vi "Lab Panel V6.00.vi"() -> ()   [LabVIEW 2017]
uses:
  sub vi/TEmp Indicator.ctl
  sub vi/SelectLAB0X-N.ctl
  sub vi/SIG LAB0X-N.ctl
  sub vi/Set LAB0X-N.ctl
  sub vi/Disp Lab.ctl
  TEmp.ctl
  <vilib>/Platform/TimedLoop/XDataNode/timing_clust.ctl
  <vilib>/Platform/TimedLoop/XDataNode/nitl_modes.ctl
  <vilib>/Platform/TimedLoop/XDataNode/wakeup.ctl
  Global 1.vi
  Global display 4.vi
  Global display 3.vi
  Global display 1.vi
  Global display 2.vi
  <vilib>/platform/TimedLoop/XDataNode/XDataNode.xnode
  <vilib>/Platform/TimedLoop/XDataNode/XDNodeRunTimeDep.lvlib
  sub vi/Web Imge control.ctl
panel:
  in  "path to JPEG file":path=path "C:/Users/Mike/Documents/Crabtree/Crabtree/Hardware/crabtree"
  out "Simulate IND":bool
  out "network error":bool
  out "TEMP":bool
  out "AI":bool
  out "Amb Temp":dbl format="%#.0f"
  out "Temp Up":dbl
  in  "stop all":bool
  in  "ADMIN":bool
  in  "Tab Control 2":T1(tab)
  out "SIG LAB05-2":T2 {"PF" format="%.2f"; "AMPS" format="%.1f"}
  out "SIG LAB05-1":T2 {"PF" format="%.2f"; "AMPS" format="%.1f"}
  out "SIG LAB04-2":T2 {"PF" format="%.2f"; "AMPS" format="%.1f"}
  out "SIG LAB04-1":T2 {"PF" format="%.2f"; "AMPS" format="%.1f"}
  out "SIG LAB03-2":T2 {"PF" format="%.2f"; "AMPS" format="%.1f"}
  out "SIG LAB03-1":T2 {"PF" format="%.2f"; "AMPS" format="%.1f"}
  out "SIG LAB02-2":T2 {"PF" format="%.2f"; "AMPS" format="%.1f"}
  in  "RUN LAB01-1":bool
  in  "O/I  LAB05-1":bool
  in  "O/I  LAB05-2":bool
  in  "O/I  LAB04-1":bool
  in  "O/I  LAB04-2":bool
  in  "O/I  LAB02-1":bool
  in  "O/I  LAB02-2":bool
  in  "O/I  LAB01-2":bool
  in  "O/I  LAB01-1":bool
  in  "O/I  LAB03-1":bool
  in  "RUN LAB05-2":bool
  in  "RUN LAB05-1":bool
  in  "RUN LAB04-2":bool
  in  "RUN LAB04-1":bool
  in  "RUN LAB03-2":bool
  in  "RUN LAB03-1":bool
  in  "RUN LAB02-2":bool
  in  "RUN LAB02-1":bool
  in  "RUN LAB01-2":bool
  in  "SELECT LAB05-2":T3
  in  "SELECT LAB05-1":T3
  in  "SELECT LAB04-2":T3
  in  "SELECT LAB04-1":T3
  in  "SELECT LAB03-2":T3
  in  "SELECT LAB03-1":T3
  in  "SELECT LAB02-2":T3
  in  "SELECT LAB02-1":T3
  in  "SELECT LAB01-2":T3
  in  "SELECT LAB01-1":T3
  in  "O/I  LAB03-2":bool
  out "SIG LAB01-1":T2 {"PF" format="%.2f"; "AMPS" format="%.1f"}
  out "SIG LAB01-2":T2 {"PF" format="%.2f"; "AMPS" format="%.1f"}
  out "SIG LAB02-1":T2 {"PF" format="%.2f"; "AMPS" format="%.1f"}
  out "DISP LAB05-2":T4 {"MINS" format="%.2g"}
  out "DISP LAB05-1":T4 {"MINS" format="%.2g"}
  out "DISP LAB04-2":T4 {"MINS" format="%.2g"}
  out "DISP LAB04-1":T4 {"MINS" format="%.2g"}
  out "DISP LAB03-2":T4 {"MINS" format="%.2g"}
  out "DISP LAB03-1":T4 {"MINS" format="%.2g"}
  in  "SET LAB05-2":T5={"NAME"="", "DESCRIPTION"="", "CYCLES"=5.0, "T-RISE mins"=0.0, "T-RISE deg C"=0.0} {"CYCLES" min=5.0 step=1.0}
  in  "SET LAB05-1":T5={"NAME"="", "DESCRIPTION"="", "CYCLES"=5.0, "T-RISE mins"=0.0, "T-RISE deg C"=0.0} {"CYCLES" min=5.0 step=1.0}
  in  "SET LAB04-2":T5={"NAME"="", "DESCRIPTION"="", "CYCLES"=5.0, "T-RISE mins"=0.0, "T-RISE deg C"=0.0} {"CYCLES" min=5.0 step=1.0}
  in  "SET LAB04-1":T5={"NAME"="", "DESCRIPTION"="", "CYCLES"=5.0, "T-RISE mins"=0.0, "T-RISE deg C"=0.0} {"CYCLES" min=5.0 step=1.0}
  in  "SET LAB03-2":T5={"NAME"="", "DESCRIPTION"="", "CYCLES"=5.0, "T-RISE mins"=0.0, "T-RISE deg C"=0.0} {"CYCLES" min=5.0 step=1.0}
  in  "SET LAB03-1":T5={"NAME"="", "DESCRIPTION"="", "CYCLES"=5.0, "T-RISE mins"=0.0, "T-RISE deg C"=0.0} {"CYCLES" min=5.0 step=1.0}
  out "DISP LAB02-2":T4 {"MINS" format="%.2g"}
  out "DISP LAB02-1":T4 {"MINS" format="%.2g"}
  in  "SET LAB02-2":T5={"NAME"="", "DESCRIPTION"="", "CYCLES"=5.0, "T-RISE mins"=0.0, "T-RISE deg C"=0.0} {"CYCLES" min=5.0 step=1.0}
  in  "SET LAB02-1":T5={"NAME"="", "DESCRIPTION"="", "CYCLES"=5.0, "T-RISE mins"=0.0, "T-RISE deg C"=0.0} {"CYCLES" min=5.0 step=1.0}
  out "RESULT LAB05-2":bool
  out "RESULT LAB05-1":bool
  out "RESULT LAB04-2":bool
  out "RESULT LAB04-1":bool
  out "RESULT LAB03-2":bool
  out "RESULT LAB03-1":bool
  out "RESULT LAB02-2":bool
  out "RESULT LAB02-1":bool
  out "RESULT LAB01-2":bool
  out "RESULT LAB01-1":bool
  in  "SET LAB01-1":T5={"NAME"="", "DESCRIPTION"="", "CYCLES"=5.0, "T-RISE mins"=0.0, "T-RISE deg C"=0.0} {"CYCLES" min=5.0 step=1.0}
  in  "SET LAB01-2":T5={"NAME"="", "DESCRIPTION"="", "CYCLES"=5.0, "T-RISE mins"=0.0, "T-RISE deg C"=0.0} {"CYCLES" min=5.0 step=1.0}
  out "DISP LAB01-1":T4 {"MINS" format="%.2g"}
  out "DISP LAB01-2":T4 {"MINS" format="%.2g"}
  out "TEMP RISE LAB05-2":cluster{"TL":dbl, "TN":dbl}
  out "TEMP RISE LAB05-1":cluster{"TL":dbl, "TN":dbl}
  out "TEMP RISE LAB04-2":cluster{"TL":dbl, "TN":dbl}
  out "TEMP RISE LAB04-1":cluster{"TL":dbl, "TN":dbl}
  out "TEMP RISE LAB03-2":cluster{"TL":dbl, "TN":dbl}
  out "TEMP RISE LAB03-1":cluster{"TL":dbl, "TN":dbl}
  out "TEMP RISE LAB02-2":cluster{"TL":dbl, "TN":dbl}
  out "TEMP RISE LAB02-1":cluster{"TL":dbl, "TN":dbl}
  out "TEMP RISE LAB01-2":cluster{"TL":dbl, "TN":dbl}
  out "TEMP RISE LAB01-1":cluster{"TL":dbl, "TN":dbl}
  out "JIG LAB05-2":bool
  out "JIG LAB05-1":bool
  out "JIG LAB04-2":bool
  out "JIG LAB04-1":bool
  out "JIG LAB03-2":bool
  out "JIG LAB03-1":bool
  out "JIG LAB02-2":bool
  out "JIG LAB02-1":bool
  out "JIG LAB01-2":bool
  out "JIG LAB01-1":bool
  out "TEMP START LAB01-1":cluster{"TL":dbl, "TN":dbl}
  out "TEMP START LAB02-1":cluster{"TL":dbl, "TN":dbl}
  out "TEMP START LAB03-1":cluster{"TL":dbl, "TN":dbl}
  out "TEMP START LAB04-1":cluster{"TL":dbl, "TN":dbl}
  out "TEMP START LAB01-2":cluster{"TL":dbl, "TN":dbl}
  out "TEMP START LAB02-2":cluster{"TL":dbl, "TN":dbl}
  out "TEMP START LAB03-2":cluster{"TL":dbl, "TN":dbl}
  out "TEMP START LAB04-2":cluster{"TL":dbl, "TN":dbl}
  out "TEMP START LAB05-2":cluster{"TL":dbl, "TN":dbl}
  out "TEMP START LAB05-1":cluster{"TL":dbl, "TN":dbl}
  out "LOG LAB05-2":string
  out "LOG LAB04-2":string
  out "LOG LAB03-2":string
  out "LOG LAB02-2":string
  out "LOG LAB01-2":string
  out "LOG LAB05-1":string
  out "LOG LAB04-1":string
  out "LOG LAB03-1":string
  out "LOG LAB02-1":string
  out "LOG LAB01-1":string
  in  "Tab charts":T6(tab)
  out "LAB01 VOLTS":dynamicdata(graph)
  out "LAB01 AMPS":dynamicdata(graph)
  out "LAB01 deg C":dynamicdata(graph)
  out "LAB02 VOLTS":dynamicdata(graph)
  out "LAB02 AMPS":dynamicdata(graph)
  out "LAB02 deg C":dynamicdata(graph)
  out "LAB03 VOLTS":dynamicdata(graph)
  out "LAB03 AMPS":dynamicdata(graph)
  out "LAB03 deg C":dynamicdata(graph)
  out "LAB04 VOLTS":dynamicdata(graph)
  out "LAB04 AMPS":dynamicdata(graph)
  out "LAB04 deg C":dynamicdata(graph)
  out "LAB05 VOLTS":dynamicdata(graph)
  out "LAB05 AMPS":dynamicdata(graph)
  out "LAB05 deg C":dynamicdata(graph)
  out "Reset Error":bool
  out "Er USB#2":dbl
  out "Er USB#1":dbl
  out "Er USB#0":dbl
  out "Resets Done":dbl
  out "Error USB #2":bool
  out "Error USB #1":bool
  out "Error USB #0":bool
  in  "MAIL SETTINGS":T7
  out "MAIL REPORT":string
  in  "TO (string):":string
  in  "Send Mail Now":bool
  in  "Auto Mail Send":bool
  in  "Network Directory":path
  in  "JIG ON TIME (S)":dbl=1.0 min=1.0 max=10.0 step=0.5 format="%.1g"
  in  "JIG OFF TIME (S)":dbl=2.0 min=2.0 max=10.0 step=0.5 format="%.1g"
  in  "Reset Measuring":bool
  out "path":path
  out "physical channels 0":string="DemoDevice,BID#0/ai0:1" caption="property value"
  out "physical channels 1":string="DemoDevice,BID#0/ai0:1" caption="property value"
  out "physical channels 2":string="DemoDevice,BID#0/ai0:1" caption="property value"
  in  "Min I":dbl=1.0
  in  "Min V":dbl=10.0
  out "JIG RELAY CYCLES":T8
  out "ON L05-2":cluster{"amps":dbl, "volts":dbl, "pf":dbl}
  out "ON L05-1":cluster{"amps":dbl, "volts":dbl, "pf":dbl}
  out "FAIL LAB05-2":cluster{"LO":dbl, "HI":dbl}
  out "FAIL LAB05-1":cluster{"LO":dbl, "HI":dbl}
  out "FAIL LAB04-2":cluster{"LO":dbl, "HI":dbl}
  out "FAIL LAB04-1":cluster{"LO":dbl, "HI":dbl}
  out "FAIL LAB03-2":cluster{"LO":dbl, "HI":dbl}
  out "FAIL LAB03-1":cluster{"LO":dbl, "HI":dbl}
  out "FAIL LAB02-2":cluster{"LO":dbl, "HI":dbl}
  out "FAIL LAB02-1":cluster{"LO":dbl, "HI":dbl}
  out "FAIL LAB01-2":cluster{"LO":dbl, "HI":dbl}
  out "FAIL LAB01-1":cluster{"LO":dbl, "HI":dbl}
  out "ON L01-1":cluster{"amps":dbl, "volts":dbl, "pf":dbl}
  out "ON L01-2":cluster{"amps":dbl, "volts":dbl, "pf":dbl}
  out "ON L02-1":cluster{"amps":dbl, "volts":dbl, "pf":dbl}
  out "ON L02-2":cluster{"amps":dbl, "volts":dbl, "pf":dbl}
  out "ON L03-1":cluster{"amps":dbl, "volts":dbl, "pf":dbl}
  out "ON L03-2":cluster{"amps":dbl, "volts":dbl, "pf":dbl}
  out "ON L04-1":cluster{"amps":dbl, "volts":dbl, "pf":dbl}
  out "ON L04-2":cluster{"amps":dbl, "volts":dbl, "pf":dbl}
  in  "Open Com Port":bool
  out "LA05-2 (TN)":bool
  out "LA05-2 (TL)":bool
  out "LA05-1 (TN)":bool
  out "LA05-1 (TL)":bool
  out "LA04-2 (TN)":bool
  out "LA04-2 (TL)":bool
  out "LA04-1 (TN)":bool
  out "LA04-1 (TL)":bool
  out "LA03-2 (TN)":bool
  out "LA03-2 (TL)":bool
  out "LA03-1 (TN)":bool
  out "LA03-1 (TL)":bool
  out "LA02-2 (TN)":bool
  out "LA02-2 (TL)":bool
  out "LA02-1 (TN)":bool
  out "LA02-1 (TL)":bool
  out "LA01-2 (TN)":bool
  out "LA01-2 (TL)":bool
  out "LA01-1 (TN)":bool
  out "LA01-1 (TL)":bool
  out "TEMP LA05":T9
  out "TEMP LA04":T9
  out "TEMP LA03":T9
  out "TEMP LA02":T9
  out "TEMP LA01":T9
  out "Ref deg C":dbl format="%#.0f"
  out "Temp read loop":dbl
  out "Com Port Status":bool
  out "Com setup loops":i32
  out "VISA Com out":refnum<visa-resource-name>
  in  "Select COM port":refnum<visa-resource-name>="COM6"
  in  "Read Temp":bool
  out "Error Temp":bool
  out "Fault Counters":u64[](array[numeric])
  out "TempErrors":bool[](array[boolean])
  in  "Temp Simulate":bool
  out "AI Task":bool
  out "AI Task2":u32
  out "AI Task1":u32
  out "AI Task0":u64
  out "Total USB resets":dbl
  in  "Auto Reset":bool
  in  "Mail Test File To:":string
  in  "Mail Test Fail":bool
  out "graph flag":bool
  in  "Temp Test Cal":dbl
  in  "Amps Fail level":dbl
  in  "Fail Loops":dbl
  out "Save JC":bool
  in  "DAQ Simulate":bool
  in  "Temp Value":dbl
  in  "Temp Delay Lps":dbl
  in  "SAMPLES":dbl
  in  "RATE (Hz)":dbl
  in  "JIG TEST":T10
  in  "C drive data root dir":path
  out "run lab05-2":bool
  out "run lab05-1":bool
  out "run lab04-2":bool
  out "run lab04-1":bool
  out "run lab03-2":bool
  out "run lab03-1":bool
  out "run lab02-2":bool
  out "run lab02-1":bool
  out "run lab01-2":bool
  out "run lab01-1":bool
  in  "Tab Control":T11(tab)
  out "LAB01-2 (GRAPH)":dynamicdata(graph)
  out "LAB01-1 (GRAPH)":dynamicdata(graph)
  out "LAB02-2 (GRAPH)":dynamicdata(graph)
  out "LAB02-1 (GRAPH)":dynamicdata(graph)
  out "LAB03-2 (GRAPH)":dynamicdata(graph)
  out "LAB03-1 (GRAPH)":dynamicdata(graph)
  out "LAB04-2 (GRAPH)":dynamicdata(graph)
  out "LAB04-1 (GRAPH)":dynamicdata(graph)
  out "LAB05-2 (GRAPH)":dynamicdata(graph)
  out "LAB05-1 (GRAPH)":dynamicdata(graph)
  out "Any Test Running":bool
  out "Read Time":dbl
  out "LAB05 TEMP":T12
  out "LAB04 TEMP":T12
  out "LAB02 TEMP":T12
  out "LAB01 TEMP":T12
  out "LAB03 TEMP":T12
  out "LAB05-TP":bool
  out "LAB04-TP":bool
  out "LAB03-TP":bool
  out "LAB02-TP":bool
  out "LAB01-TP":bool
  out "Analog error":bool
  out "USB OUT 0":bool[](array[boolean])
  out "USB OUT 1":bool[](array[boolean])
  out "USB OUT 2":bool[](array[boolean])
  in  "Ambient Volts":dbl format="%.2f"
  in  "PF":dbl min=0.0 max=1.0 step=0.1 format="%#.1f"
  in  "VOLTS":dbl
  in  "OFF amps":dbl min=0.0 max=100.0 step=0.1 format="%#.1f"
  in  "ON amps":dbl
  in  "LAB deg C":T13
  out "AI data 0":waveform(dbl)[](array[waveform])
  out "AI data 1":waveform(dbl)[](array[waveform])
  out "AI data 2":waveform(dbl)[](array[waveform])
  out "AI Error":errorcluster[](array[cluster])
  out "error array":errorcluster[](array[cluster])
  out "AI loop time":dbl format="%.6g"
  out "loops":dbl
  out "on loops":dbl format="%#.0f"
  out "off loops":dbl format="%#.0f"
  out "jig cycle":dbl
  out "TDMS LAB01-1":refnum<k34>
  out "data file error":errorcluster
  out "TDMS LAB02-1":refnum<k34>
  out "TDMS LAB01-2":refnum<k34>
  out "TDMS LAB02-2":refnum<k34>
  out "TDMS LAB03-1":refnum<k34>
  out "TDMS LAB03-2":refnum<k34>
  out "TDMS LAB04-1":refnum<k34>
  out "TDMS LAB04-2":refnum<k34>
  out "TDMS LAB05-1":refnum<k34>
  out "TDMS LAB05-2":refnum<k34>
  out "mail control":string
  out "File Time Stamp":timestamp
  in  "stop":bool
  out "deg C (volts)":dbl
  out "Application Directory":path
  out "ACQ Init TIme":u32
  out "ACQ Time":u32
  out "Web Server:Root Directory Path":path
  out "Analog Fault Counts":i32[](array[numeric])
  out "Timed loop Finished Late":bool
  in  "Set Loop Time":T14=500.0 format="%#_13g"
  out "Loop Time":u32
  out "Process AIs":bool
  in  "DigOutDelay":u32=5
  out "TEMP REF cal":dbl
  out "CAL LAB01":T15 {"2 (TN) cal" min=0.0 step=0.01 format="%.2f"; "2 (TL) cal" min=0.0 step=0.01 format="%.2f"; "2 (PF) cal" min=0.0 step=0.01 format="%.2f"; "2 (V) cal" min=0.0 step=0.01 format="%.2f"; "2 (A) cal" min=0.0 step=0.01 format="%.2f"; "1 (TN) cal" min=0.0 step=0.01 format="%.2f"; "1 (TL) cal" min=0.0 step=0.01 format="%.2f"; "1 (PF) cal" min=0.0 step=0.01 format="%.2f"; "1 (V) cal" min=0.0 step=0.01 format="%.2f"; "1  (A) cal" min=0.0 step=0.01 format="%.2f"}
  out "CAL LAB03":T15 {"2 (TN) cal" min=0.0 step=0.01 format="%.2f"; "2 (TL) cal" min=0.0 step=0.01 format="%.2f"; "2 (PF) cal" min=0.0 step=0.01 format="%.2f"; "2 (V) cal" min=0.0 step=0.01 format="%.2f"; "2 (A) cal" min=0.0 step=0.01 format="%.2f"; "1 (TN) cal" min=0.0 step=0.01 format="%.2f"; "1 (TL) cal" min=0.0 step=0.01 format="%.2f"; "1 (PF) cal" min=0.0 step=0.01 format="%.2f"; "1 (V) cal" min=0.0 step=0.01 format="%.2f"; "1  (A) cal" min=0.0 step=0.01 format="%.2f"}
  out "CAL LAB02":T16 {"2 (TN) cal" min=0.0 step=0.01 format="%.2f"; "2 (TL) cal" min=0.0 step=0.01 format="%.2f"; "2 (PF) cal" min=0.0 step=0.01 format="%.2f"; "2 (V) cal" min=0.0 step=0.01 format="%.2f"; "2 (A) cal" min=0.0 step=0.01 format="%.2f"; "1 (TN) cal" min=0.0 step=0.01 format="%.2f"; "1 (TL) cal" min=0.0 step=0.01 format="%.2f"; "1 (PF) cal" min=0.0 step=0.01 format="%.2f"; "1 (V) cal" min=0.0 step=0.01 format="%.2f"; "1 (A) cal" min=0.0 step=0.01 format="%.2f"}
  out "CAL LAB04":T15 {"2 (TN) cal" min=0.0 step=0.01 format="%.2f"; "2 (TL) cal" min=0.0 step=0.01 format="%.2f"; "2 (PF) cal" min=0.0 step=0.01 format="%.2f"; "2 (V) cal" min=0.0 step=0.01 format="%.2f"; "2 (A) cal" min=0.0 step=0.01 format="%.2f"; "1 (TN) cal" min=0.0 step=0.01 format="%.2f"; "1 (TL) cal" min=0.0 step=0.01 format="%.2f"; "1 (PF) cal" min=0.0 step=0.01 format="%.2f"; "1 (V) cal" min=0.0 step=0.01 format="%.2f"; "1  (A) cal" min=0.0 step=0.01 format="%.2f"}
  out "cal file error out":errorcluster
  in  "SET (cal)":bool
  out "LAB05 (CAL)":T15 {"2 (TN) cal" min=0.0 step=0.01 format="%.2f"; "2 (TL) cal" min=0.0 step=0.01 format="%.2f"; "2 (PF) cal" min=0.0 step=0.01 format="%.2f"; "2 (V) cal" min=0.0 step=0.01 format="%.2f"; "2 (A) cal" min=0.0 step=0.01 format="%.2f"; "1 (TN) cal" min=0.0 step=0.01 format="%.2f"; "1 (TL) cal" min=0.0 step=0.01 format="%.2f"; "1 (PF) cal" min=0.0 step=0.01 format="%.2f"; "1 (V) cal" min=0.0 step=0.01 format="%.2f"; "1  (A) cal" min=0.0 step=0.01 format="%.2f"}
  out "LAB05":T17
  out "x-y":dbl
  out "x*y":dbl
  out "OFF amps 2":dbl
  out "Lab05 -1 Offset I":dbl
  out "AI Data 0":waveform(dbl)[](graph)
  out "AI Data 1":waveform(dbl)[](graph)
  out "AI Data 2":waveform(dbl)[](graph)
  # "v6.36"
  # "LAB01"
  # "LAB02"
  # "LAB03"
  # "LAB04"
  # "LAB05"
  # "LAB01"
  # "LAB02"
  # "LAB03"
  # "LAB04"
  # "LAB05"
  # "PANEL ID / DATE / TIME / NAME / DESCRIPTION / CYCLES / TEST TIME / STATUS"
  # "PANEL ID / DATE / TIME / NAME / DESCRIPTION / CYCLES / TEST TIME / STATUS"
  # "http://This IP:8000/Lab_Panel"
  # "(Enter recipients address seperated by comma)"
  # "JIG SET"
  # "Temperature circuits \ndetected at start up."
  # "PANEL CONTROL TO BE ON"
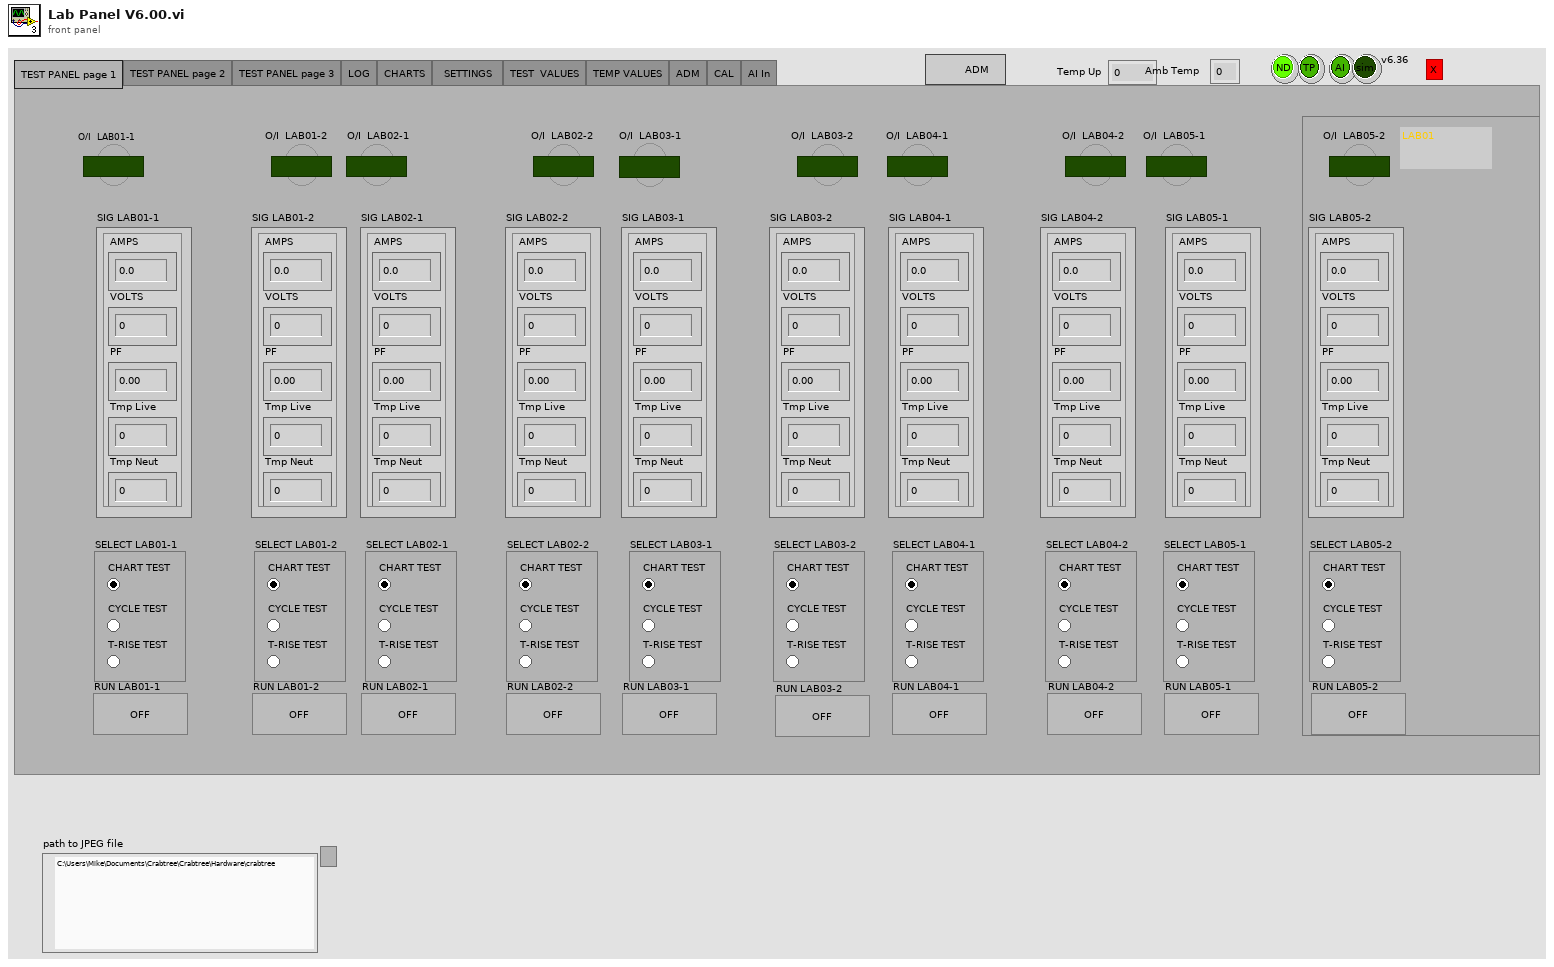
[diagram p1: front panel]
types:
  T1 = enum32{"TEST PANEL page 1", "TEST PANEL page 2", "TEST PANEL page 3", "LOG", "CHARTS", "SETTINGS   ", "TEST  VALUES", "TEMP VALUES", "ADM", "CAL", "AI In"}
  T2 = typedef "SIG LAB0X-N.ctl" = cluster{"AMPS":dbl, "VOLTS":dbl, "PF":dbl, "Tmp Live":dbl, "Tmp Neut":dbl}
  T3 = typedef "SelectLAB0X-N.ctl" = enum32{"CHART TEST", "CYCLE TEST", "T-RISE TEST"}
  T4 = typedef "Disp Lab.ctl" = cluster{"CYCLE":dbl, "MINS":dbl, "STATUS":string}
  T5 = typedef "Set LAB0X-N.ctl" = cluster{"NAME":string, "DESCRIPTION":string, "CYCLES":dbl, "T-RISE mins":dbl, "T-RISE deg C":dbl}
  T6 = enum32{"LAB01", "LAB02", "LAB03", "LAB04", "LAB05"}
  T7 = cluster{"OUT SERVER ADDRESS":string, "FROM ACCOUNT":string, "USER NAME":string, "PASSWORD":string, "TEST MAIL":bool, "TEST MAIL STATUS":string, "mail error":errorcluster}
  T8 = cluster{"LAB01-1":dbl, "LAB01-2":dbl, "LAB02-1":dbl, "LAB02-2":dbl, "LAB03-1":dbl, "LAB03-2":dbl, "LAB04-1":dbl, "LAB04-2":dbl, "LAB05-1":dbl, "LAB05-2":dbl}
  T9 = cluster{"TL-1":dbl, "TN-1":dbl, "TL-2":dbl, "TN-2":dbl, "TL -1COUNT":dbl, "TN-1 COUNT":dbl, "TL-2 COUNT":dbl, "TN-2 COUNT":dbl}
  T10 = cluster{" LAB01-1":bool, " LAB01-2":bool, "LAB02-1":bool, " LAB02-2":bool, "LAB03-1":bool, "LAB03-2":bool, "LAB04-1":bool, "LAB04-2":bool, "LAB05-1":bool, "LAB05-2":bool}
  T11 = enum32{"LAB01", "LAB02", "LAB03", "LAB04", "LAB05", "TEMPERATURE", "GENERAL INFO", "Simulate", "AI Data Out", "AI Init"}
  T12 = typedef "TEmp Indicator.ctl" = cluster{"T1 Live":dbl, "T1 Neut":dbl, "T2 Live":dbl, "T2 Neut":dbl, "ID":dbl, "ER":dbl}
  T13 = cluster{"1 TL":dbl, "1 TN":dbl, "2 TL":dbl, "2 TN":dbl, "ID":dbl, "ER":dbl}
  T14 = typedef "TEmp.ctl" = dbl
  T15 = cluster{"1  (A) cal":dbl, "1 (V) cal":dbl, "1 (PF) cal":dbl, "1 (TL) cal":dbl, "1 (TN) cal":dbl, "2 (A) cal":dbl, "2 (V) cal":dbl, "2 (PF) cal":dbl, "2 (TL) cal":dbl, "2 (TN) cal":dbl}
  T16 = cluster{"1 (A) cal":dbl, "1 (V) cal":dbl, "1 (PF) cal":dbl, "1 (TL) cal":dbl, "1 (TN) cal":dbl, "2 (A) cal":dbl, "2 (V) cal":dbl, "2 (PF) cal":dbl, "2 (TL) cal":dbl, "2 (TN) cal":dbl}
  T17 = cluster{"LAB05-1 (A)":dbl, "LAB05-1 (V)":dbl, "LAB05-1 (PF)":dbl, "LAB05-2 (A)":dbl, "LAB05-2 (V)":dbl, "LAB05-2 (PF)":dbl}
  T18 = enum8{"Enabled", "Disabled", "Disabled and Grayed Out"}
  T19 = enum16{"open", "replace", "create", "open or create", "replace or create", "replace or create with confirmation"}
  T20 = typedef "XDNodeRunTimeDep.lvlib/timing_clust.ctl" = cluster{"Expected End [f-1]":u64, "Actual End [f-1]":u64, "Finished Late? [f-1]":bool, "Expected End [i-1]":u64, "Actual End [i-1]":u64, "Finished Late? [i-1]":bool, "Expected Start [i]":u64, "Actual Start [i]":u64, "Expected Start [f]":u64, "Actual Start [f]":u64, "Source Name":string, "Structure Name":string, "Period":i64, "Deadline":i64, "Offset":i64, "Start":i64, "Priority":i32, "Timeout":i32, "Mode":T21, "Wakeup Reason":T22, "Error":errorcluster, "Source Type":string, "Secondary Source Type":string, "Global End Time":u64, "Global Start Time":u64, "Frame Duration":u64, "Iteration Duration":u64, "Assigned CPU":i32, "I/O Scan Engine Mode":u32}
  T21 = typedef "XDNodeRunTimeDep.lvlib/nitl_modes.ctl" = enum32{"No Change", "Process missed periods, maintain original phase", "Discard missed periods, maintain original phase", "Process missed periods, ignore original phase", "Discard missed periods, ignore original phase"}
  T22 = typedef "XDNodeRunTimeDep.lvlib/wakeup.ctl" = enum32{"Normal", "Aborted", "Asynchronous wakeup", "Timing source error", "Timed loop error", "Timeout"}
  T23 = enum16{"open", "open or create", "create or replace", "create", "open (read-only)"}
  T24 = cluster{"status":string, "mail server":string, "mail from":string, "mail to":string, "mail file":bool}
  T25 = typedef "Web Imge control.ctl" = cluster{"Tab Ref":refnum<vi>, "Values":i32[]}
  T26 = cluster{"SET LAB01-1":T5, "SET LAB01-2":T5, "SET LAB02-1":T5, "SET LAB02-2":T5, "SET LAB03-1":T5, "SET LAB03-2":T5, "SET LAB04-1":T5, "SET LAB04-2":T5, "SET LAB05-1":T5, "SET LAB05-2":T5, "Network Directory":path, "C drive data root dir":path, "RATE (Hz)":dbl, "SAMPLES":dbl, "Select COM port":refnum<visa-resource-name>, "Temp Delay Lps":dbl, "Temp Value":dbl, "Fail Loops":dbl, "Temp Test Cal":dbl, "Amps Fail level":dbl, "Mail Test File To:":string, "Mail Test Fail":bool, "Set Loop Time":T14, "DigOutDelay":u32}
  T27 = cluster{"MAIL SETTINGS":cluster{"OUT SERVER ADDRESS":string, "FROM ACCOUNT":string, "USER NAME":string, "PASSWORD":string, "TEST MAIL":bool, "TEST MAIL STATUS":string, "mail error":errorcluster}, "Auto Mail Send":bool, string}
  T28 = cluster{"T1 Live":dbl, "T1 Neut":dbl, "T2 Live":dbl, "T2 Neut":dbl, "ID":dbl, "ER":dbl}
  T29 = cluster{"id1":bool, "id2":bool, "id3":bool, "id4":bool, "id5":bool}
  T30 = cluster{"T1":dbl, "T2":dbl, "T3":dbl, "T4":dbl, "ID":dbl, "ER":dbl}
  T31 = typedef "imagedata.ctl" = cluster{"image type":i32, "image depth":i32, "image":u8[], "mask":u8[], "colors":u32[], "Rectangle":cluster{"left":i16, "top":i16, "right":i16, "bottom":i16}}
  T32 = cluster{"STATUS":string, "OUT SERVER ADDRESS":string, "FROM ACCOUNT":string, "Mail Test File To:":string, "Mail Test Fail":bool}
  T33 = cluster{"LAB01-1 (A)":dbl, "LAB01-1 (V)":dbl, "LAB01-1 (PF)":dbl, "LAB01-2 (A)":dbl, "LAB01-2 (V)":dbl, "LAB01-2 (PF)":dbl}
  T34 = cluster{"LAB02-1 (A)":dbl, "LAB02-1 (V)":dbl, "LAB02-1 (PF)":dbl, "LAB02-2 (A)":dbl, "LAB02-2 (V)":dbl, "LAB02-2 (PF)":dbl}
  T35 = cluster{"LAB03-1 (A)":dbl, "LAB03-1 (V)":dbl, "LAB03-1 (PF)":dbl, "LAB03-2 (A)":dbl, "LAB03-2 (V)":dbl, "LAB03-2 (PF)":dbl}
  T36 = cluster{"LAB04-1 (A)":dbl, "LAB04-1 (V)":dbl, "LAB04-1 (PF)":dbl, "LAB04-2 (A)":dbl, "LAB04-2 (V)":dbl, "LAB04-2 (PF)":dbl}
  T37 = cluster{"OFF amps":dbl, "VOLTS":dbl, "PF":dbl, "OFF amps":dbl, "VOLTS":dbl, "PF":dbl}
  T38 = cluster{"1  (A) cal":dbl, "1 (V) cal":dbl, "1 (PF) cal":dbl, "1 (TL) cal":dbl, "1 (TN) cal":dbl, "2 (A) cal":dbl, "2 (V) cal":dbl, "2 (PF) cal":dbl, "2 (TL) cal":dbl, "2 (TN) cal":dbl, "1  (A)Zero Offset":dbl, "2  (A)Zero Offset 1":dbl}
  T39 = cluster{"FAIL LAB01-1":cluster{"LO":dbl, "HI":dbl}, "SIG LAB01-1":T2, "TEMP START LAB01-1":cluster{"TL":dbl, "TN":dbl}, "DISP LAB01-1":T4, "SET LAB01-1":T5, "TDMS LAB01-1":refnum<k34>}
  T40 = cluster{"CYCLE":dbl, "MINS":dbl, "STATUS":string}
  T41 = cluster{"FAIL LAB01-2":cluster{"LO":dbl, "HI":dbl}, "SIG LAB01-2":T2, "TEMP START LAB01-2":cluster{"TL":dbl, "TN":dbl}, "DISP LAB01-2":T4, "SET LAB01-2":T5, "TDMS LAB01-2":refnum<k34>}
  T42 = cluster{"FAIL LAB02-1":cluster{"LO":dbl, "HI":dbl}, "SIG LAB02-1":T2, "TEMP START LAB02-1":cluster{"TL":dbl, "TN":dbl}, "DISP LAB02-1":T4, "SET LAB02-1":T5, "TDMS LAB02-1":refnum<k34>}
  T43 = cluster{"FAIL LAB02-2":cluster{"LO":dbl, "HI":dbl}, "SIG LAB02-2":T2, "TEMP START LAB02-2":cluster{"TL":dbl, "TN":dbl}, "DISP LAB02-2":T4, "SET LAB02-2":T5, "TDMS LAB02-2":refnum<k34>}
  T44 = cluster{"FAIL LAB03-1":cluster{"LO":dbl, "HI":dbl}, "SIG LAB03-1":T2, "TEMP START LAB03-1":cluster{"TL":dbl, "TN":dbl}, "DISP LAB03-1":T4, "SET LAB03-1":T5, "TDMS LAB03-1":refnum<k34>}
  T45 = cluster{"FAIL LAB03-2":cluster{"LO":dbl, "HI":dbl}, "SIG LAB03-2":T2, "TEMP START LAB03-2":cluster{"TL":dbl, "TN":dbl}, "DISP LAB03-2":T4, "SET LAB03-2":T5, "TDMS LAB03-2":refnum<k34>}
  T46 = cluster{"FAIL LAB04-1":cluster{"LO":dbl, "HI":dbl}, "SIG LAB04-1":T2, "TEMP START LAB04-1":cluster{"TL":dbl, "TN":dbl}, "DISP LAB04-1":T4, "SET LAB04-1":T5, "TDMS LAB04-1":refnum<k34>}
  T47 = cluster{"FAIL LAB04-2":cluster{"LO":dbl, "HI":dbl}, "SIG LAB04-2":T2, "TEMP START LAB04-2":cluster{"TL":dbl, "TN":dbl}, "DISP LAB04-2":T4, "SET LAB04-2":T5, "TDMS LAB04-2":refnum<k34>}
  T48 = cluster{"FAIL LAB05-1":cluster{"LO":dbl, "HI":dbl}, "SIG LAB05-1":T2, "TEMP START LAB05-1":cluster{"TL":dbl, "TN":dbl}, "DISP LAB05-1":T4, "SET LAB05-1":T5, "TDMS LAB05-1":refnum<k34>}
  T49 = cluster{"FAIL LAB05-2":cluster{"LO":dbl, "HI":dbl}, "SIG LAB05-2":T2, "TEMP START LAB05-2":cluster{"TL":dbl, "TN":dbl}, "DISP LAB05-2":T4, "SET LAB05-2":T5, "TDMS LAB05-2":refnum<k34>}
  T50 = cluster{"MAIL SETTINGS":cluster{"OUT SERVER ADDRESS":string, "FROM ACCOUNT":string, "USER NAME":string, "PASSWORD":string, "TEST MAIL":bool, "TEST MAIL STATUS":string, "mail error":errorcluster}, "Auto Mail Send":bool, "TO (string):":string}
  T51 = cluster{"TP1-L":dbl, "TP1-N":dbl, "TP2-L":dbl, "TP2-N":dbl, "TP1-L COUNT":dbl, "TP1-N COUNT":dbl, "TP2-L COUNT":dbl, "TP2-N COUNT":dbl}
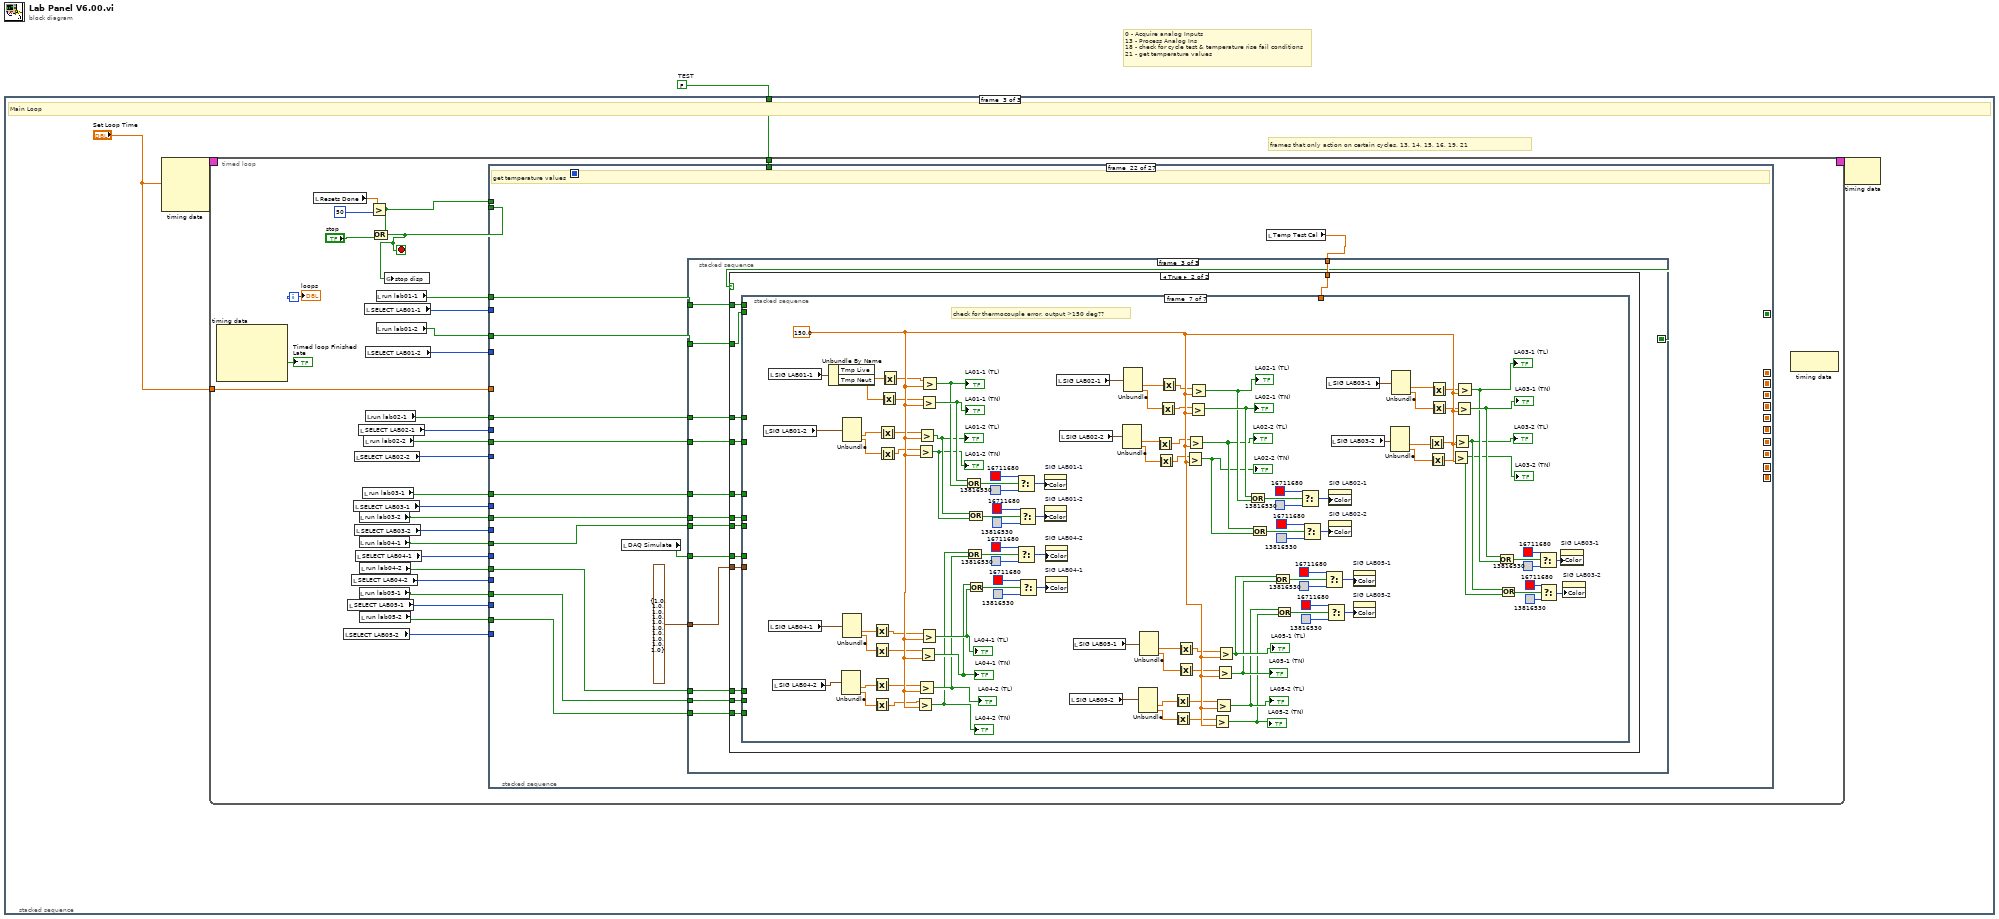
[diagram p0: block diagram]
diagram:
  w1 = FALSE  # TEST
  # "0 - Acquire analog Inputs\n13 - Process Analog Ins\n18 - check for cycle test & temperature rise fail conditions\n21 - get temperature values"
  n1 = stacked-sequence {
    tunnel: w1 -> [_ w12 w354]
    frame #0 {
      # "Front panel Terminals (???)"
      n2 = local write "Save JC"(FALSE) -> ()
      n3 = call "App Data Files and folders.vi"("ApplicationName"="Crabtree LabPanel" ("name or relative path")) -> ("Exec Log Path"=w3:path)  [unwired: 8 in, 2 out]
      n4 = call "ExecLog_CreateLog.vi"("Enable"=TRUE, "file path"=w3) -> ()  [unwired: 4 in, 3 out]
      n5 = disable-structure shown="Disabled" {
        frame Disabled {
          n6 = Open Application Reference() -> (3:w11:refnum<vi>)  [unwired: 4 in, 1 out]
          n7 = property class="App"(reference=w11, "WebSrvr.Active"=TRUE ("Web Server:Server Active")) -> (reference out=w10:refnum<vi>, error out=w7:errorcluster, "WebSrvr.RootPath"=→"Web Server:Root Directory Path":path)  [unwired: 1 in]
          n8 = Close Reference(reference=w10) -> ()  [unwired: 1 in, 1 out]
          n9 = call <vilib>:"Simple Error Handler.vi"("error in (no error)"=w7) -> ()  [unwired: 4 in, 5 out]
        }
        frame Enabled {
        }
      }
      "jig cycle" <- 0
    }
    frame #1 {
      # "do 1st time set up"
      n10 = stacked-sequence {
        tunnel: w12 -> [_ w15 _ _ _ _ _ _ _ _ _ w337 _ _]
        frame #0 {
          # "check for simulate mode"
          n11 = call "subvi-simulate v1.vi"() -> ("Sim"=w13:bool)  [unwired: 11 in]
          n12 = case shown="True" w13 {
            frame False {
            }
            frame True {
              w14 = TRUE
              n13 = local write "Temp Simulate"(w14) -> ()
              n14 = local write "DAQ Simulate"(w14) -> ()
            }
          }
        }
        frame #1 {
          # "RESET USB AND TEMPERATURE CIRCUITS"
          n15 = local read "DAQ Simulate"() -> (w16:bool)
          n16 = case shown="False" w16 {
            tunnel: w15 -> [w17 _]
            frame False {
              n17 = call "Reset USB&temp v 1.vi"("Test"=w17) -> ()  [unwired: 10 in, 1 out]
            }
            frame True {
            }
          }
        }
        frame #2 {
          # "Disable front panel while 1st time set up is being done         -                Configure Web Server"
          n18 = disable-structure shown="Enabled" {
            frame Enabled {
              n19 = property on="Tab Control 2" class="TabCtl (strict)"() -> ("Pages"=w35:refnum<vi>[])  [unwired: 2 in, 2 out]
              n20 = Index Array(array=w35, index=8) -> (element=w33:refnum<vi>)
              n21 = property class="Page"(reference=w33, "PageVis"=FALSE) -> ()  [unwired: 1 in, 2 out]
            }
            frame Disabled {
            }
          }
          n22 = property on="Tab Control 2" class="TabCtl (strict)"("Value"=0) -> ()  [unwired: 2 in, 2 out]
          n23 = local write "ADMIN"(FALSE) -> ()
          n24 = property on="Tab Control 2" class="TabCtl (strict)"("DisabledEnum"=T18."Disabled and Grayed Out" ("Disabled")) -> ()  [unwired: 2 in, 2 out]
          n25 = call <vilib>:"Application Directory.vi"() -> ("Application Directory"=w18:path)
          n26 = Call Chain() -> (call chain=w21:string[])
          n27 = Current VI's Path() -> (path=→"path":path)
          n28 = Array Size(array=w21) -> (size(s)=w23:i32)
          n29 = Open Application Reference() -> (3:w28:refnum<vi>)  [unwired: 4 in, 1 out]
          n30 = Decrement(x=w23) -> (x-1=w22:i32)
          n31 = Index Array(array=w21, index=w22) -> (element=w20:string)
          n32 = Build Path(base path=w18, name or relative path=w20) -> (appended path=→"Application Directory":path)
          n33 = property class="App"(reference=w28, "WebSrvr.Active"=TRUE ("Web Server:Server Active"), "WebSrvr.RootPath"=w18) -> (reference out=w26:refnum<vi>, error out=w24:errorcluster)  [unwired: 1 in]
          n34 = Close Reference(reference=w26) -> ()  [unwired: 1 in, 1 out]
          n35 = call <vilib>:"Simple Error Handler.vi"("error in (no error)"=w24) -> ()  [unwired: 4 in, 5 out]
        }
        frame #3 {
          # "Get calibration values"
          n36 = call "sub vi - get calibration values v1.vi"() -> ("TEMP REF CAL"=w37:dbl, "LAB01 (CAL)"=→"CAL LAB01":T15, "LAB02 (CAL)"=→"CAL LAB02":T16, "LAB03 (CAL)"=→"CAL LAB03":T15, "LAB04 (CAL)"=→"CAL LAB04":T15, "calibration file error out"=→"cal file error out":errorcluster, "LAB05 (CAL)"=→"LAB05 (CAL)":T15)  [unwired: 9 in]
          n37 = local write "TEMP REF cal"(w37) -> ()
        }
        frame #4 {
          # "get last saved test settings from file"
          n38 = local read "Network Directory"() -> (w69:path)
          n39 = local read "C drive data root dir"() -> (w67:path)
          n40 = local read "SET LAB05-2"() -> (w99:T5)
          n41 = local read "SAMPLES"() -> (w65:dbl)
          n42 = local read "SET LAB05-1"() -> (w100:T5)
          n43 = local read "RATE (Hz)"() -> (w66:dbl)
          n44 = local read "SET LAB04-2"() -> (w101:T5)
          n45 = local read "SET LAB03-2"() -> (w98:T5)
          n46 = local read "SET LAB04-1"() -> (w102:T5)
          n47 = local read "SET LAB03-1"() -> (w97:T5)
          n48 = local read "SET LAB02-2"() -> (w96:T5)
          n49 = local read "SET LAB02-1"() -> (w95:T5)
          n50 = local read "SET LAB01-2"() -> (w94:T5)
          n51 = local read "SET LAB01-1"() -> (w93:T5)
          n52 = local read "Select COM port"() -> (w62:refnum<visa-resource-name>)
          n53 = local read "Temp Delay Lps"() -> (w61:dbl)
          n54 = local read "Mail Test File To:"() -> (w51:string)
          n55 = local read "Temp Value"() -> (w60:dbl)
          n56 = local read "Set Loop Time"() -> (w46:T14)
          n57 = local read "Temp Test Cal"() -> (w55:dbl)
          n58 = local read "Amps Fail level"() -> (w54:dbl)
          n59 = local read "DigOutDelay"() -> (w45:u32)
          n60 = local read "Fail Loops"() -> (w57:dbl)
          n61 = local read "Mail Test Fail"() -> (w49:bool)
          n62 = Bundle("SET LAB01-1"=w93, "SET LAB01-2"=w94, "SET LAB02-1"=w95, "SET LAB02-2"=w96, "SET LAB03-1"=w97, "SET LAB03-2"=w98, "SET LAB04-1"=w102, "SET LAB04-2"=w101, "SET LAB05-1"=w100, "SET LAB05-2"=w99, "Network Directory"=w69, "C drive data root dir"=w67, "RATE (Hz)"=w66, "SAMPLES"=w65, "Select COM port"=w62, "Temp Delay Lps"=w61, "Temp Value"=w60, "Fail Loops"=w57, "Temp Test Cal"=w55, "Amps Fail level"=w54, "Mail Test File To:"=w51, "Mail Test Fail"=w49, "Set Loop Time"=w46, "DigOutDelay"=w45) -> (w86:T26)  [unwired: 1 in]
          n63 = String To Path(string="c:\\crabtree\\Set Up\\") -> (path=w90:path)
          n64 = Build Path(base path=w90, name or relative path="settings.bin") -> (appended path=w88:path)
          n65 = Create Folder(path (use dialog)=w90) -> (error out=w92:errorcluster)  [unwired: 2 in, 2 out]
          n66 = call <vilib>:"Clear Errors.vi"("error in (no error)"=w92) -> ()  [unwired: 5 in, 2 out]
          n67 = Open/Create/Replace File(file path (use dialog)=w88) -> (refnum out=w85:refnum<file>, error out=w87:errorcluster)  [unwired: 5 in, 1 out]
          n68 = Read from Binary File(5:w86, 8:w87, 11:w85) -> (0:w82:errorcluster, 2:w84:T26, 3:w83:refnum<file>)  [unwired: 3 in, 1 out]
          n69 = Unbundle(w84) -> ("SET LAB01-1"=w80:T5, "SET LAB01-2"=w79:T5, "SET LAB02-1"=w78:T5, "SET LAB02-2"=w77:T5, "SET LAB03-1"=w76:T5, "SET LAB03-2"=w75:T5, "SET LAB04-1"=w74:T5, "SET LAB04-2"=w73:T5, "SET LAB05-1"=w72:T5, "SET LAB05-2"=w71:T5, "Network Directory"=w70:path, "C drive data root dir"=w68:path, "RATE (Hz)"=w63:dbl, "SAMPLES"=w64:dbl, "Select COM port"=w47:refnum<visa-resource-name>, "Temp Delay Lps"=w59:dbl, "Temp Value"=w58:dbl, "Fail Loops"=w56:dbl, "Temp Test Cal"=w53:dbl, "Amps Fail level"=w52:dbl, "Mail Test File To:"=w50:string, "Mail Test Fail"=w48:bool, "Set Loop Time"=w44:T14, "DigOutDelay"=w43:u32)
          n70 = Close File(refnum=w83, error in=w82) -> (error out=w81:errorcluster)  [unwired: 1 out]
          n71 = local write "data file error"(w81) -> ()
          n72 = local write "SET LAB05-2"(w71) -> ()
          n73 = local write "Network Directory"(w70) -> ()
          n74 = local write "C drive data root dir"(w68) -> ()
          n75 = local write "RATE (Hz)"(w63) -> ()
          n76 = local write "SAMPLES"(w64) -> ()
          n77 = local write "Select COM port"(w47) -> ()
          n78 = global write "Global 1.vi" "COM port"(w47) -> ()
          n79 = local write "Temp Delay Lps"(w59) -> ()
          n80 = local write "Temp Value"(w58) -> ()
          n81 = local write "Fail Loops"(w56) -> ()
          n82 = local write "Temp Test Cal"(w53) -> ()
          n83 = local write "Amps Fail level"(w52) -> ()
          n84 = local write "Mail Test File To:"(w50) -> ()
          n85 = local write "Mail Test Fail"(w48) -> ()
          n86 = local write "Set Loop Time"(w44) -> ()
          n87 = local write "DigOutDelay"(w43) -> ()
          n88 = local write "SET LAB04-2"(w73) -> ()
          n89 = local write "SET LAB05-1"(w72) -> ()
          n90 = local write "SET LAB04-1"(w74) -> ()
          n91 = local write "SET LAB02-1"(w78) -> ()
          n92 = local write "SET LAB02-2"(w77) -> ()
          n93 = local write "SET LAB03-1"(w76) -> ()
          n94 = local write "SET LAB03-2"(w75) -> ()
          n95 = local write "SET LAB01-1"(w80) -> ()
          n96 = local write "SET LAB01-2"(w79) -> ()
        }
        frame #5 {
          # "Get total resets value from file"
          n97 = String To Path(string="c:\\crabtree\\Set Up\\") -> (path=w113:path)
          n98 = Build Path(base path=w113, name or relative path="USB resets.bin") -> (appended path=w106:path)
          n99 = Create Folder(path (use dialog)=w113) -> (error out=w105:errorcluster)  [unwired: 2 in, 2 out]
          n100 = call <vilib>:"Clear Errors.vi"("error in (no error)"=w105) -> ()  [unwired: 5 in, 2 out]
          n101 = Open/Create/Replace File(file path (use dialog)=w106, operation (0:open)=T19."open or create") -> (refnum out=w111:refnum<file>, error out=w110:errorcluster)  [unwired: 4 in, 1 out]
          n102 = local read "Total USB resets"() -> (w104:dbl)
          n103 = Read from Binary File(5:w104, 8:w110, 11:w111) -> (0:w108:errorcluster, 2:w103:dbl, 3:w109:refnum<file>)  [unwired: 3 in, 1 out]
          n104 = local write "Total USB resets"(w103) -> ()
          n105 = Close File(refnum=w109, error in=w108) -> (error out=w107:errorcluster)  [unwired: 1 out]
          n106 = local write "data file error"(w107) -> ()
        }
        frame #6 {
          # "Get last saved jig cycles value from file"
          n107 = String To Path(string="c:\\crabtree\\Jig Cycles\\") -> (path=w125:path)
          n108 = Build Path(base path=w125, name or relative path="jigcycles.bin") -> (appended path=w123:path)
          n109 = Create Folder(path (use dialog)=w125) -> (error out=w127:errorcluster)  [unwired: 2 in, 2 out]
          n110 = call <vilib>:"Clear Errors.vi"("error in (no error)"=w127) -> ()  [unwired: 5 in, 2 out]
          n111 = Open/Create/Replace File(file path (use dialog)=w123) -> (refnum out=w121:refnum<file>, error out=w122:errorcluster)  [unwired: 5 in, 1 out]
          n112 = Read from Binary File(5:T8 {"LAB01-1"=0.0, "LAB01-2"=0.0, "LAB02-1"=0.0, "LAB02-2"=0.0, "LAB03-1"=0.0, "LAB03-2"=0.0, "LAB04-1"=0.0, "LAB04-2"=0.0, "LAB05-1"=0.0, "LAB05-2"=0.0} ("JIG RELAY CYCLES"), 8:w122, 11:w121) -> (0:w119:errorcluster, 2:w116:T8, 3:w120:refnum<file>)  [unwired: 3 in, 1 out]
          n113 = local write "JIG RELAY CYCLES"(w116) -> ()
          n114 = Close File(refnum=w120, error in=w119) -> (error out=w118:errorcluster)  [unwired: 1 out]
          n115 = local write "data file error"(w118) -> ()
        }
        frame #7 {
          # "Get mail settings"
          n116 = local read "Auto Mail Send"() -> (w131:bool)
          n117 = local read "MAIL SETTINGS"() -> (w135:T7)
          n118 = String To Path(string="c:\\crabtree\\Set Up\\") -> (path=w143:path)
          n119 = Build Path(base path=w143, name or relative path="mail.bin") -> (appended path=w141:path)
          n120 = Create Folder(path (use dialog)=w143) -> (error out=w145:errorcluster)  [unwired: 2 in, 2 out]
          n121 = Bundle("MAIL SETTINGS"=w135, "Auto Mail Send"=w131, "") -> (w134:T27)  [unwired: 1 in]
          n122 = call <vilib>:"Clear Errors.vi"("error in (no error)"=w145) -> ()  [unwired: 5 in, 2 out]
          n123 = Open/Create/Replace File(file path (use dialog)=w141) -> (refnum out=w139:refnum<file>, error out=w140:errorcluster)  [unwired: 5 in, 1 out]
          n124 = Read from Binary File(5:w134, 8:w140, 11:w139) -> (0:w137:errorcluster, 2:w133:T27, 3:w138:refnum<file>)  [unwired: 3 in, 1 out]
          n125 = Close File(refnum=w138, error in=w137) -> (error out=w136:errorcluster)  [unwired: 1 out]
          n126 = local write "data file error"(w136) -> ()
          n127 = Unbundle(w133) -> ("MAIL SETTINGS"=w132:T7, "Auto Mail Send"=w130:bool, w129:string)
          n128 = local write "Auto Mail Send"(w130) -> ()
          n129 = local write "TO (string):"(w129) -> ()
          n130 = local write "MAIL SETTINGS"(w132) -> ()
        }
        frame #8 {
          # "Set display status if blank"
          n131 = local read "DISP LAB03-2"() -> (w175:T4)
          n132 = local read "DISP LAB03-1"() -> (w182:T4)
          n133 = local read "DISP LAB02-2"() -> (w189:T4)
          n134 = local read "DISP LAB01-2"() -> (w202:T4)
          n135 = local read "DISP LAB01-1"() -> (w211:T4)
          n136 = local read "DISP LAB02-1"() -> (w196:T4)
          n137 = Unbundle(w175) -> ("STATUS"=w177:string)  [unwired: 2 out]
          n138 = Unbundle(w182) -> ("STATUS"=w184:string)  [unwired: 2 out]
          n139 = Unbundle(w189) -> ("STATUS"=w191:string)  [unwired: 2 out]
          n140 = Unbundle(w196) -> ("STATUS"=w198:string)  [unwired: 2 out]
          n141 = Unbundle(w202) -> ("STATUS"=w205:string)  [unwired: 2 out]
          n142 = Unbundle(w211) -> ("STATUS"=w212:string)  [unwired: 2 out]
          n143 = Equal?(x="", y=w177) -> (x = y?=w179:bool)
          n144 = Equal?(x="", y=w184) -> (x = y?=w186:bool)
          n145 = Equal?(x="", y=w191) -> (x = y?=w193:bool)
          n146 = Equal?(x="", y=w198) -> (x = y?=w200:bool)
          n147 = Equal?(x="", y=w205) -> (x = y?=w207:bool)
          n148 = Equal?(x="", y=w212) -> (x = y?=w214:bool)
          n149 = Select(t="STOP", s=w179, f=w177) -> (s? t:f=w176:string)
          n150 = Select(t="STOP", s=w186, f=w184) -> (s? t:f=w183:string)
          n151 = Select(t="STOP", s=w193, f=w191) -> (s? t:f=w190:string)
          n152 = Select(t="STOP", s=w200, f=w198) -> (s? t:f=w197:string)
          n153 = Select(t="STOP", s=w207, f=w205) -> (s? t:f=w204:string)
          n154 = Select(t="STOP", s=w214, f=w212) -> (s? t:f=w210:string)
          n155 = Bundle(cluster=w175, "STATUS"=w176) -> (w174:T4)  [unwired: 2 in]
          n156 = Bundle(cluster=w182, "STATUS"=w183) -> (w181:T4)  [unwired: 2 in]
          n157 = Bundle(cluster=w189, "STATUS"=w190) -> (w188:T4)  [unwired: 2 in]
          n158 = Bundle(cluster=w196, "STATUS"=w197) -> (w195:T4)  [unwired: 2 in]
          n159 = Bundle(cluster=w202, "STATUS"=w204) -> (w203:T4)  [unwired: 2 in]
          n160 = Bundle(cluster=w211, "STATUS"=w210) -> (w209:T4)  [unwired: 2 in]
          n161 = local write "DISP LAB01-2"(w203) -> ()
          n162 = local write "DISP LAB01-1"(w209) -> ()
          n163 = local write "DISP LAB02-1"(w195) -> ()
          n164 = local write "DISP LAB03-1"(w181) -> ()
          n165 = local write "DISP LAB02-2"(w188) -> ()
          n166 = local write "DISP LAB03-2"(w174) -> ()
          n167 = local read "DISP LAB05-2"() -> (w147:T4)
          n168 = local read "DISP LAB05-1"() -> (w154:T4)
          n169 = local read "DISP LAB04-2"() -> (w156:T4)
          n170 = local read "DISP LAB04-1"() -> (w158:T4)
          n171 = Unbundle(w147) -> ("STATUS"=w149:string)  [unwired: 2 out]
          n172 = Unbundle(w154) -> ("STATUS"=w160:string)  [unwired: 2 out]
          n173 = Unbundle(w156) -> ("STATUS"=w165:string)  [unwired: 2 out]
          n174 = Unbundle(w158) -> ("STATUS"=w170:string)  [unwired: 2 out]
          n175 = Equal?(x="", y=w149) -> (x = y?=w151:bool)
          n176 = Equal?(x="", y=w160) -> (x = y?=w162:bool)
          n177 = Equal?(x="", y=w165) -> (x = y?=w167:bool)
          n178 = Equal?(x="", y=w170) -> (x = y?=w172:bool)
          n179 = Select(t="STOP", s=w151, f=w149) -> (s? t:f=w148:string)
          n180 = Select(t="STOP", s=w162, f=w160) -> (s? t:f=w159:string)
          n181 = Select(t="STOP", s=w167, f=w165) -> (s? t:f=w164:string)
          n182 = Select(t="STOP", s=w172, f=w170) -> (s? t:f=w169:string)
          n183 = Bundle(cluster=w147, "STATUS"=w148) -> (w146:T4)  [unwired: 2 in]
          n184 = Bundle(cluster=w154, "STATUS"=w159) -> (w153:T4)  [unwired: 2 in]
          n185 = Bundle(cluster=w156, "STATUS"=w164) -> (w155:T4)  [unwired: 2 in]
          n186 = Bundle(cluster=w158, "STATUS"=w169) -> (w157:T4)  [unwired: 2 in]
          n187 = local write "DISP LAB05-2"(w146) -> ()
          n188 = local write "DISP LAB05-1"(w153) -> ()
          n189 = local write "DISP LAB04-1"(w157) -> ()
          n190 = local write "DISP LAB04-2"(w155) -> ()
        }
        frame #9 {
          w219 = 0
          w216 = FALSE
          # "initialise analog error control"
          n191 = local write "Resets Done"(0) -> ()
          n192 = local write "Auto Reset"(TRUE) -> ()
          n193 = local write "Er USB#0"(w219) -> ()
          n194 = local write "Er USB#1"(w219) -> ()
          n195 = local write "Er USB#2"(w219) -> ()
          n196 = local write "Analog error"(w216) -> ()
          n197 = local write "Reset Measuring"(w216) -> ()
          n198 = local write "Error USB #0"(w216) -> ()
          n199 = local write "Reset Error"(w216) -> ()
          n200 = local write "Error USB #1"(w216) -> ()
          n201 = local write "Error USB #2"(w216) -> ()
          n202 = local write "stop"(w216) -> ()
          n203 = local write "stop all"(w216) -> ()
        }
        frame #10 {
          # "get initial temperature values"
          n204 = stacked-sequence {
            frame #0 {
              w228 = T28 {"T1 Live"=20.0, "T1 Neut"=20.0, "T2 Live"=20.0, "T2 Neut"=20.0, "ID"=6.0, "ER"=10.0} ("LAB01 TEMP")
              n205 = local read "Select COM port"() -> (w223:refnum<visa-resource-name>)
              n206 = local write "LAB deg C"(w228) -> ()
              n207 = global write "Global display 4.vi" "LAB deg C"(w228) -> ()
              n208 = local write "OFF amps"(1.5) -> ()
              n209 = local write "ON amps"(20.0) -> ()
              n210 = local write "VOLTS"(250.0) -> ()
              n211 = local write "PF"(0.5) -> ()
